vi "Receive and Prepare Messages Live.vi"(10 "Notifiers":T1) -> (0 "error out":errorcluster, 1 "params":variant, 2 "message":string, 3 "LSM Run Live":refnum<notifier>)   [LabVIEW 2020]
uses:
  _Controls/Notifiers.ctl
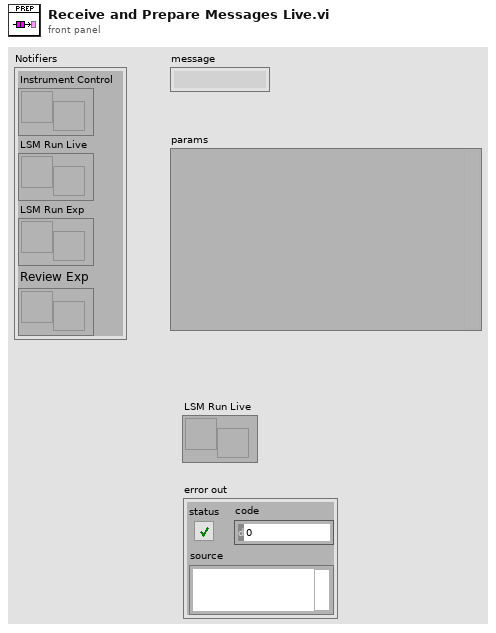
[diagram p1: front panel]
types:
  T1 = typedef "Notifiers.ctl" = cluster{"Instrument Control":refnum<notifier>, "LSM Run Live":refnum<notifier>, "LSM Run Exp":refnum<notifier>, "Review Exp":refnum<notifier>}
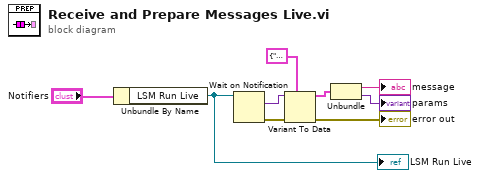
[diagram p0: block diagram]
diagram:
  n1 = Unbundle By Name("Notifiers") -> ("LSM Run Live"=w6:refnum<notifier>)
  "LSM Run Live" <- w6
  n2 = Wait on Notification(notifier=w6) -> (notification=w4:variant, error out=w7:errorcluster)  [unwired: 3 in, 2 out]
  n3 = Variant To Data(error in=w7, type=cluster{"message":string, "params":variant} {"message"="", "params"=variant} ("output cluster"), Variant=w4) -> (data=w2:cluster{"message":string, "params":variant}, error out=→"error out":errorcluster)
  n4 = Unbundle(w2) -> ("message"=→"message":string, "params"=→"params":variant)
